vi "contPIDantiWindup.vi"(4 "Saturation M":dbl, 6 "Saturation U":dbl, 8 "PID Gains":cluster{"Kp":dbl, "Kd":dbl, "Ki":dbl, "Ts":dbl}={"Kp"=0.0, "Kd"=0.0, "Ki"=0.0, "Ts"=1.0}, 10 "Position":dbl, 11 "Reference":dbl) -> (3 "control":dbl)   [LabVIEW 2011, in "kevLib2011.lvlib"]
uses:
  kevLib2011.lvlib
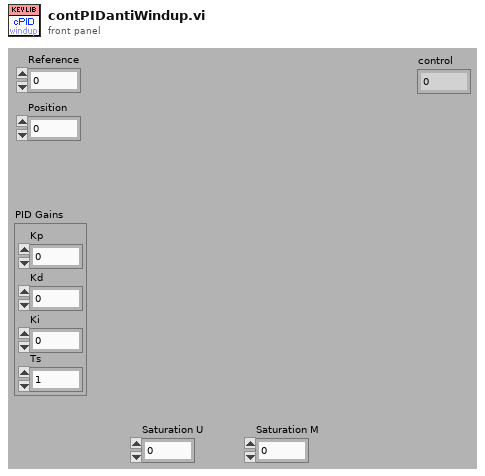
[diagram p1: front panel]
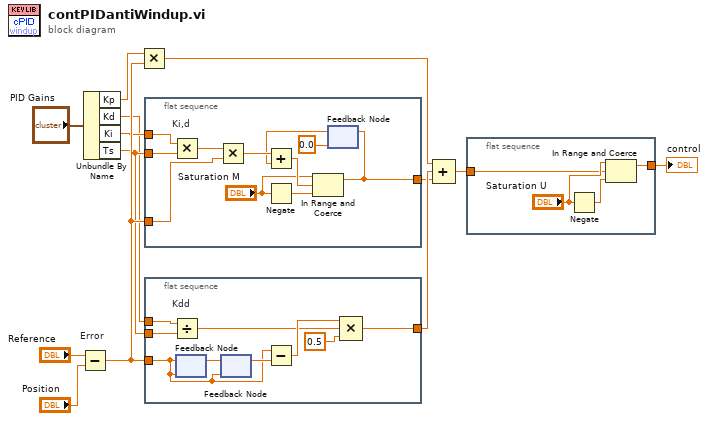
[diagram p0: block diagram]
diagram:
  n1 = Subtract "Error"(x="Reference", y="Position") -> (x-y=w6:dbl)
  n2 = Unbundle By Name("PID Gains") -> ("Kp"=w10:dbl, "Kd"=w3:dbl, "Ki"=w5:dbl, "Ts"=w4:dbl)
  n3 = Multiply(x=w10, y=w6) -> (x*y=w9:dbl)
  n4 = flat-sequence {
    tunnel: [w14] -> w7
    tunnel: w6 -> [w23]
    tunnel: w5 -> [w20]
    tunnel: w4 -> [w18]
    frame #0 {
      n5 = Multiply "Ki,d"(x=w20, y=w18) -> (x*y=w19:dbl)
      n6 = Multiply(x=w19, y=w23) -> (x*y=w22:dbl)
      n7 = Negate(x="Saturation M") -> (-x=w15:dbl)
      n8 = feedback #1(0.0 ("value")) -> (w21:dbl)
      n9 = Add(x=w22, y=w21) -> (x+y=w17:dbl)
      n10 = In Range and Coerce(upper limit="Saturation M", x=w17, lower limit=w15) -> (coerced(x)=w14:dbl)  [unwired: 1 out]
      n11 = feedback-in #1(w14) -> ()
    }
  }
  n12 = flat-sequence {
    tunnel: [w29] -> w8
    tunnel: w6 -> [w28]
    tunnel: w4 -> [w27]
    tunnel: w3 -> [w26]
    frame #0 {
      n13 = Divide "Kdd"(x=w26, y=w27) -> (x/y=w25:dbl)
      n14 = feedback #2(w28) -> (w33:dbl)
      n15 = feedback-in #2(w28) -> ()
      n16 = feedback #3(w28) -> (w32:dbl)
      n17 = feedback-in #3(w33) -> ()
      n18 = Subtract(x=w28, y=w32) -> (x-y=w31:dbl)
      n19 = Compound Arithmetic op=MULTIPLY(w31, w25, 0.5 ("value")) -> (w29:dbl)
    }
  }
  n20 = Compound Arithmetic op=ADD(w9, w8, w7) -> (w2:dbl)
  n21 = flat-sequence {
    tunnel: w2 -> [w35]
    tunnel: [w34] -> w1
    frame #0 {
      n22 = Negate(x="Saturation U") -> (-x=w36:dbl)
      n23 = In Range and Coerce(upper limit="Saturation U", x=w35, lower limit=w36) -> (coerced(x)=w34:dbl)  [unwired: 1 out]
    }
  }
  "control" <- w1
